vi "Solve2.vi"(8 "Error In":errorcluster, 11 "object in":refnum<class "2024_13.lvclass">) -> (0 "Error Out":errorcluster, 2 "Result":u64, 3 "object out":refnum<class "2024_13.lvclass">)   [LabVIEW 2023, in "2024_13.lvclass"]
uses:
  2024_13.lvclass
  2024_13.lvclass/2024_13.ctl
  <vilib>/Analysis/7linalg.llb/Solve Linear Equations (single right hand).vi
  <vilib>/Analysis/baseanly.llb/Solve Linear Equations By Cholesky.vi
  <vilib>/Analysis/baseanly.llb/Real Matrix to Compact Array.vi
  <vilib>/Analysis/baseanly.llb/Real Compact Tri-Matrix Linear Eqs.vi
  <vilib>/Analysis/7linalg.llb/Solve Linear Eqs (General).vi
  <vilib>/Analysis/7linalg.llb/Solve Linear Eqs (Gen, single right hand).vi
  <vilib>/Analysis/NI_AALPro.lvlib
panel:
  out "Result 2":u64
  out "Array":dbl[](array[numeric])
  out "Solution Vector":dbl[](array[numeric]) format="%.2f"
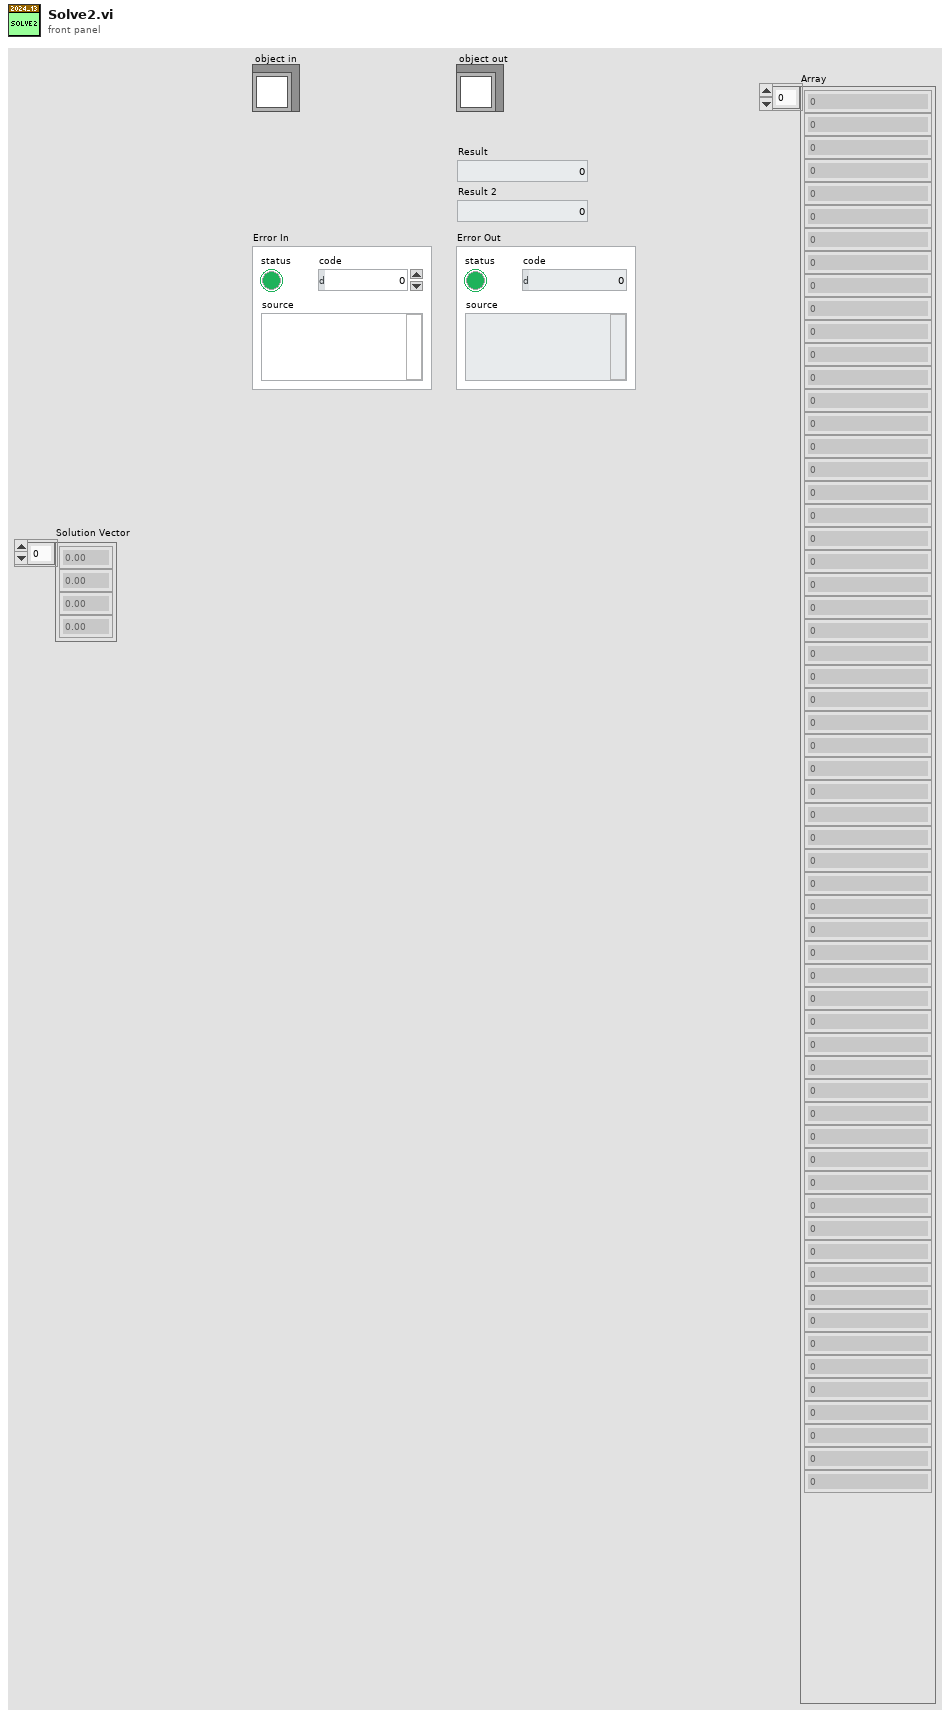
[diagram p1: front panel]
types:
  T1 = typedef "2024_13.lvclass/Game.ctl" = cluster{"A":T2, "B":T2, "Prize":T2}
  T2 = typedef "AOC_XY.ctl" = cluster{"X":u64, "Y":u64}
  T3 = typedef "NI_Matrix.lvlib/RealMatrix.ctl" = dbl[][]
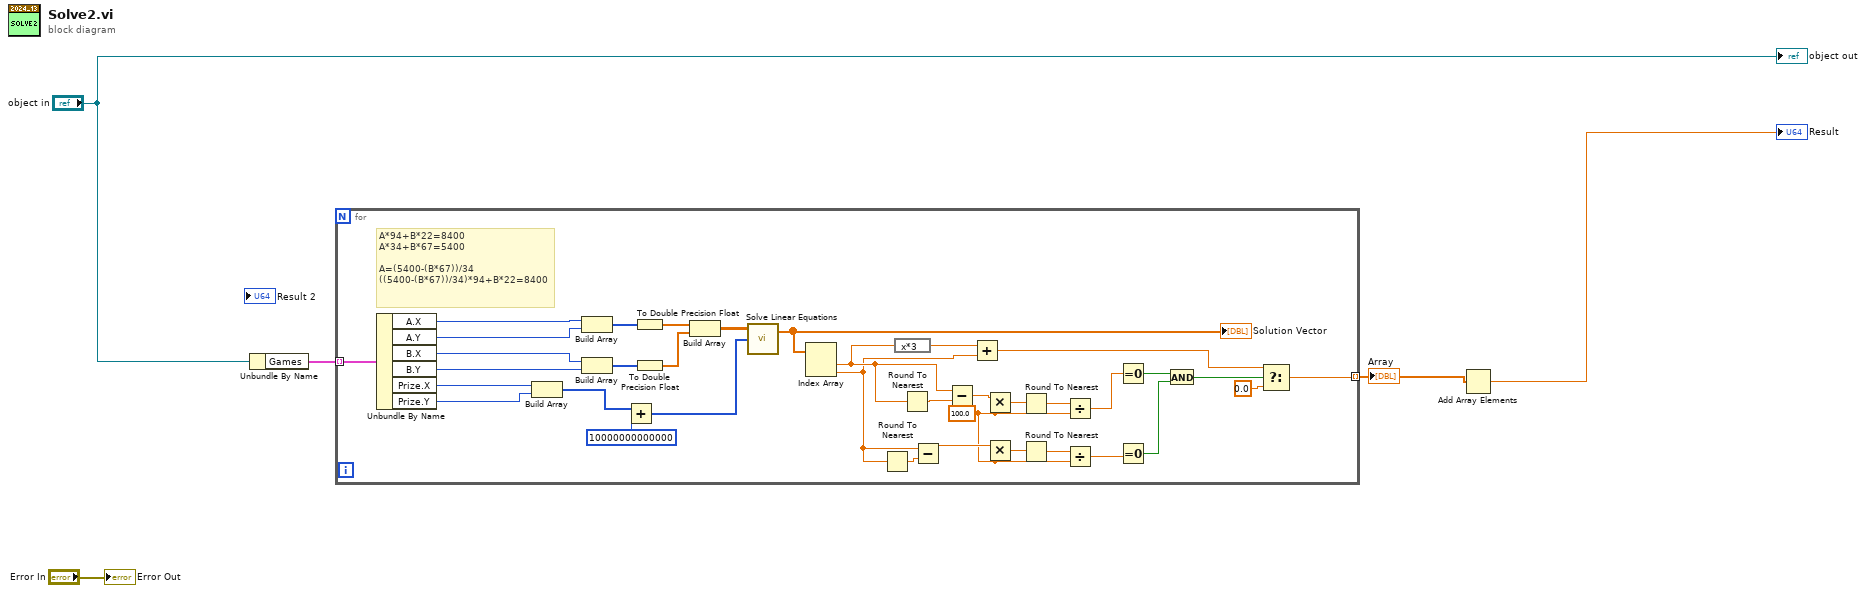
[diagram p0: block diagram]
diagram:
  n1 = Unbundle By Name("object in") -> ("Games"=w3:T1[])
  n2 = for {
    tunnel: w3 -> [w41] mode=indexing
    tunnel: [w22] -> w2 mode=indexing
    w10 = 100.0 ("y")
    # "A*94+B*22=8400\nA*34+B*67=5400\n\nA=(5400-(B*67))/34\n((5400-(B*67))/34)*94+B*22=8400"
    n3 = Unbundle By Name(w41) -> ("A.X"=w40:u64, "A.Y"=w31:u64, "B.X"=w30:u64, "B.Y"=w39:u64, "Prize.X"=w33:u64, "Prize.Y"=w32:u64)
    n4 = Build Array(w33, w32) -> (w7:u64[])
    n5 = Build Array(w40, w31) -> (w38:u64[])
    n6 = Build Array(w30, w39) -> (w37:u64[])
    n7 = Add(x=w7, y=u64 10000000000000) -> (x+y=w6:u64[])
    n8 = To Double Precision Float(number=w38) -> (double precision float=w36:dbl[])
    n9 = To Double Precision Float(number=w37) -> (double precision float=w35:dbl[])
    n10 = Build Array(w36, w35) -> (w34:T3)
    n11 = call-poly <vilib>:"Solve Linear Equations.vi"("Known Vector"=w6, "Input Matrix"=w34) -> ("Solution Vector"=w29:dbl[])  [unwired: 1 in, 1 out]
    "Solution Vector" <- w29
    n12 = Index Array(array=w29) -> (element #1=w19:dbl, element #2=w18:dbl)  [unwired: 2 in]
    n13 = Round To Nearest(number=w18) -> (nearest integer value=w20:dbl)
    n14 = expression code="x*3"(w19) -> (w28:dbl)
    n15 = Round To Nearest(number=w19) -> (nearest integer value=w21:dbl)
    n16 = Subtract(x=w18, y=w20) -> (x-y=w11:dbl)
    n17 = Subtract(x=w19, y=w21) -> (x-y=w17:dbl)
    n18 = Add(x=w28, y=w18) -> (x+y=w24:dbl)
    n19 = Multiply(x=w17, y=w10) -> (x*y=w16:dbl)
    n20 = Multiply(x=w11, y=w10) -> (x*y=w12:dbl)
    n21 = Round To Nearest(number=w16) -> (nearest integer value=w15:dbl)
    n22 = Round To Nearest(number=w12) -> (nearest integer value=w13:dbl)
    n23 = Divide(x=w15, y=w10) -> (x/y=w14:dbl)
    n24 = Divide(x=w13, y=w10) -> (x/y=w9:dbl)
    n25 = Equal To 0?(x=w14) -> (x = 0?=w27:bool)
    n26 = Equal To 0?(x=w9) -> (x = 0?=w26:bool)
    n27 = And(x=w27, y=w26) -> (x .and. y?=w25:bool)
    n28 = Select(t=w24, s=w25, f=0.0 ("y")) -> (s? t:f=w22:dbl)
  }
  "Array" <- w2
  n29 = Add Array Elements(numeric array=w2) -> (sum=→"Result":dbl)
  "Error Out" <- "Error In"
  "object out" <- "object in"
